vi "niRFUtil MT UTIL WF Error Handler.vi"(0 "path to calling VI":path, 1 "dt":dbl, 9 "waveform length (samples)":i32, 11 "error in (no error)":errorcluster) -> (6 "error?":bool, 15 "error out":errorcluster)   [LabVIEW 2015, in "niRFUtil.lvlib"]
uses:
  niRFUtil.lvlib
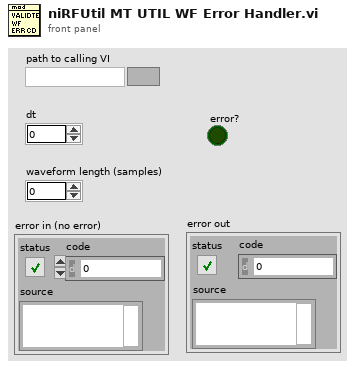
[diagram p1: front panel]
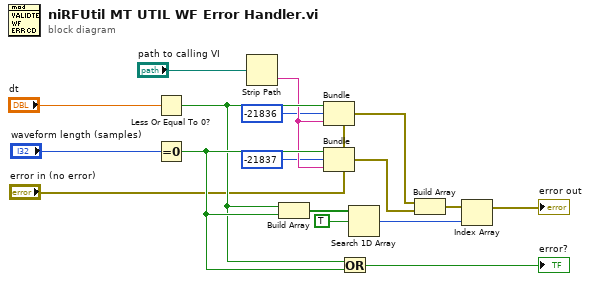
[diagram p0: block diagram]
diagram:
  n1 = Less Or Equal To 0?(x="dt") -> (x <= 0?=w15:bool)
  n2 = Equal To 0?(x="waveform length (samples)") -> (x = 0?=w16:bool)
  n3 = Strip Path(path="path to calling VI") -> (name=w8:string)  [unwired: 1 out]
  n4 = Build Array(w15, w16) -> (w4:bool[])
  n5 = Bundle(cluster="error in (no error)", "status"=w15, "code"=-21836, "source"=w8) -> (w9:errorcluster)
  n6 = Bundle(cluster="error in (no error)", "status"=w16, "code"=-21837, "source"=w8) -> (w10:errorcluster)
  n7 = Or(x=w15, y=w16) -> (x .or. y?=→"error?":bool)
  n8 = Search 1D Array(1D array=w4, element=TRUE) -> (index of element=w3:i32)  [unwired: 1 out]
  n9 = Build Array(w9, w10) -> (w6:errorcluster[])
  n10 = Index Array(array=w6, index=w3) -> (element=→"error out":errorcluster)
